vi "_AllThingsCLI.vi"   [LabVIEW 2022 SP3]
types:
  T1 = typedef "ArduinoCtrl.ctl" = cluster{"CLI directory":path, "Connection":string[], "Code Directory":path}
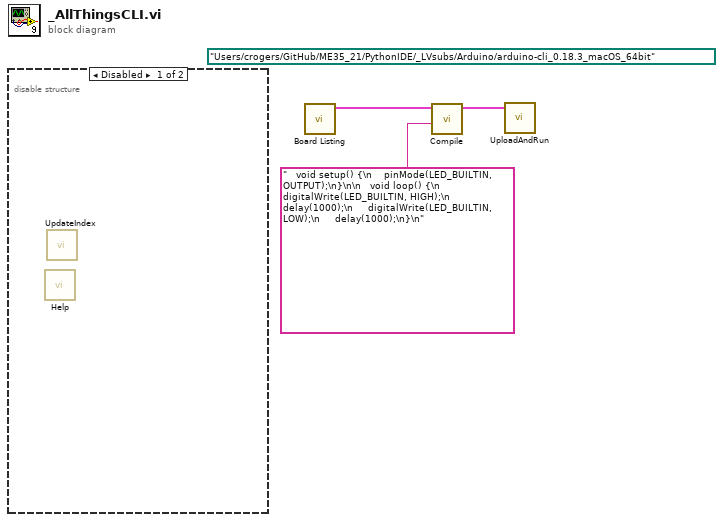
[diagram p0: block diagram]
diagram:
  (unwired) path "/Users/crogers/GitHub/ME35_21/PythonIDE/_LVsubs/Arduino/arduino-cli_0.18.3_macOS_64bit" ("CLI directory")
  n1 = disable-structure shown="Disabled" {
    frame Disabled {
      n2 = call "Help.vi"() -> ()  [unwired: 12 in]
      n3 = call "UpdateIndex.vi"() -> ()  [unwired: 12 in]
    }
    frame Enabled {
    }
  }
  n4 = call "Board Listing.vi"() -> ("Arduino"=w3:T1)  [unwired: 9 in, 2 out]
  n5 = call "Compile.vi"("Code"="   void setup() {\n    pinMode(LED_BUILTIN, OUTPUT);\n}\n\n   void loop() {\n     digitalWrite(LED_BUILTIN, HIGH);\n     delay(1000);\n     digitalWrite(LED_BUILTIN, LOW);\n     delay(1000);\n}\n", "Arduino in"=w3) -> ("Arduino out"=w1:T1)  [unwired: 6 in, 3 out]
  n6 = call "UploadAndRun.vi"("Arduino in"=w1) -> ()  [unwired: 7 in, 4 out]
